vi "Do.vi"(8 "error in":errorcluster, 10 "Actor in":refnum<class "Actor.lvclass">, 11 "Update Device Config MSG":refnum<class "Update Device Config MSG.lvclass">) -> (0 "error out":errorcluster, 2 "Actor out":refnum<class "Actor.lvclass">)   [LabVIEW 2017, in "Controller.lvlib" / "Update Device Config MSG.lvclass"]
doc: "(<B>Filename</B>: Actor Framework.lvlib:Message.lvclass:Do.vi)\n\nDefines what a message does when it is received by an actor. Generally, a message instructs an actor to invoke one of its methods. By default, this method does nothing. A child class must override it to define behavior. Create a child class by using the Actor Framework Message Maker dialog box."
uses:
  Update Device Config MSG.lvclass
  C:/Program Files (x86)/National Instruments/LabVIEW 2017/vi.lib/MSR Consulting, LLC/Devices/DAQ Device/Messages/Device Configuration/Get Serialized Device Configuration MSG.lvclass
  <vilib>/ActorFramework/Actor/Actor.lvclass
  <vilib>/MSR Consulting, LLC/General Reuse/SuperActor/SuperActor.lvclass
  C:/Program Files (x86)/National Instruments/LabVIEW 2017/vi.lib/ActorFramework/Actor/Actor.lvclass
  <vilib>/MSR Consulting, LLC/Devices/DAQ Device/Messages/Device Configuration/Get Serialized Device Configuration MSG.lvclass/Get Serialized Device Configuration MSG.ctl
  <vilib>/MSR Consulting, LLC/General Reuse/SuperActor/SuperActor.lvclass/SuperActor.ctl
  <vilib>/MSR Consulting, LLC/Devices/DAQ Device/Messages/Device Configuration/Read cfg cluster.vi
  <vilib>/MSR Consulting, LLC/General Reuse/SuperActor/Read CVT Session.vi
  <vilib>/MSR Consulting, LLC/General Reuse/SuperActor/Read Log Session.vi
  <vilib>/MSR Consulting, LLC/General Reuse/Session APIs/_Session Fwk/Session - Root.lvclass
  <vilib>/MSR Consulting, LLC/General Reuse/Session APIs/CVT/CVT.lvclass
  <vilib>/MSR Consulting, LLC/General Reuse/Session APIs/Session Log/System Log.lvclass
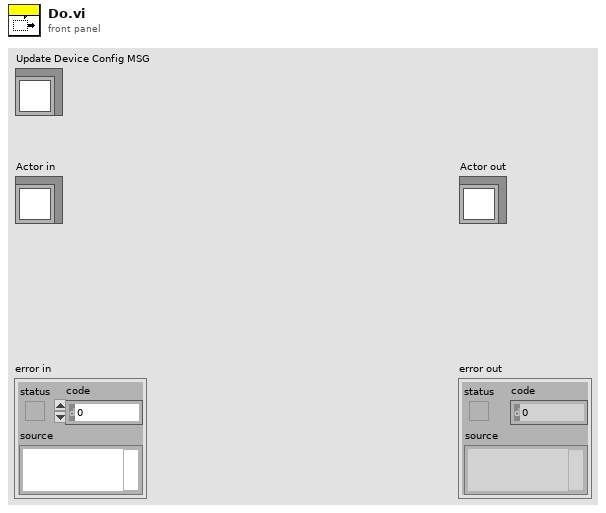
[diagram p1: front panel]
types:
  T1 = typedef "DAQ Device.lvlib/Cfg Msg.ctl" = cluster{"ID":string, "type":string, "label":string, "SN":string, "controller_":bool, "Addr":string, "Model":string, "Device Active":bool}
  T2 = typedef "Session - Root.lvclass/Session Handle.ctl" = refnum<data-value>
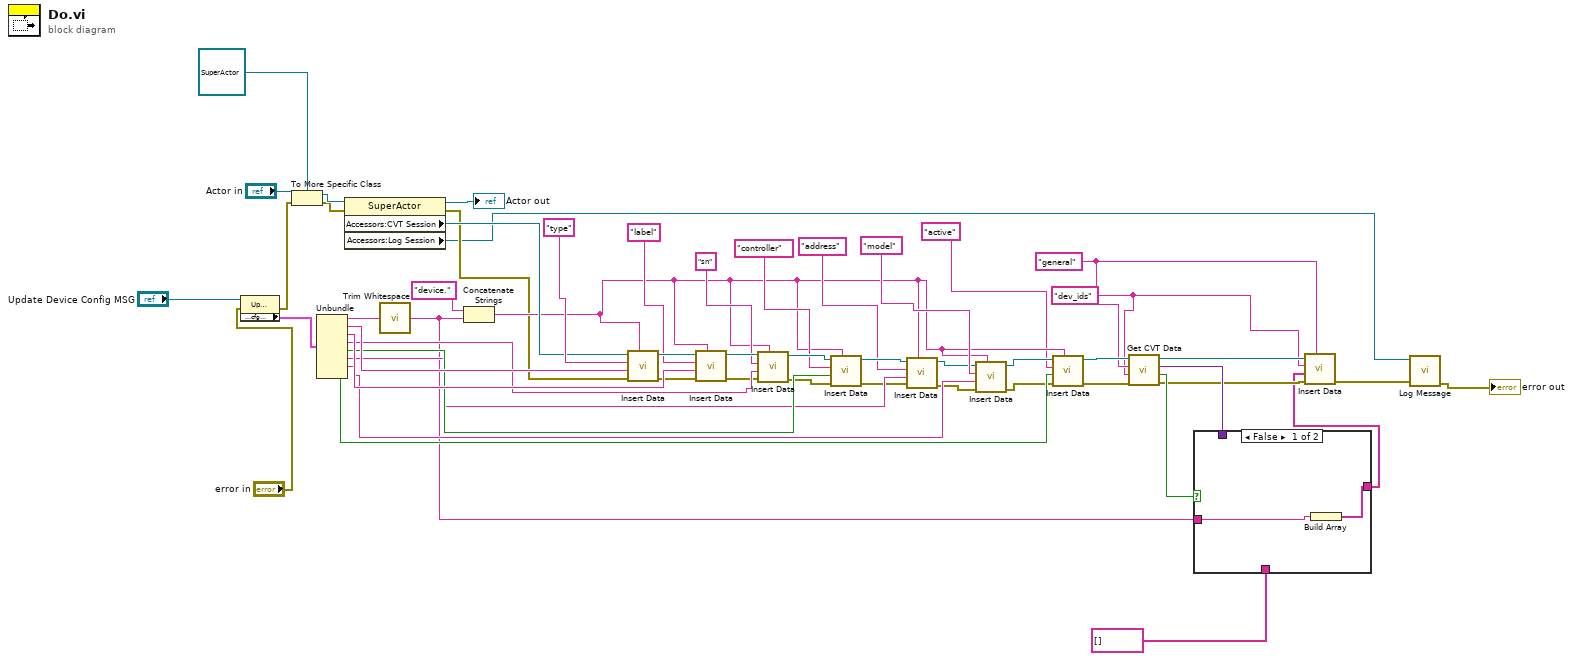
[diagram p0: block diagram]
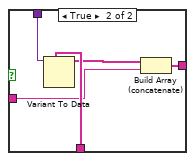
[diagram p2: hidden frame]
diagram:
  w2 = "general" ("Group")
  w1 = "dev_ids" ("Group")
  n1 = property class="Update Device Config MSG.lvclas"(reference="Update Device Config MSG", error in="error in") -> (error out=w23:errorcluster, "Accessors:cfg cluster"=w49:T1)  [unwired: 1 out]
  n2 = To More Specific Class(target class=refnum<class "SuperActor.lvclass"> refnum ("SuperActor.lvlib:SuperActor"), reference="Actor in", error in=w23) -> (specific class reference=w52:refnum<class "SuperActor.lvclass">, error out=w22:errorcluster)
  n3 = Unbundle(w49) -> ("ID"=w47:string, "type"=w44:string, "label"=w41:string, "SN"=w38:string, "controller_"=w35:bool, "Addr"=w32:string, "Model"=w29:string, "Device Active"=w25:bool)
  n4 = property class="SuperActor"(reference=w52, error in=w22) -> (reference out=→"Actor out":refnum<class "SuperActor.lvclass">, error out=w21:errorcluster, "Accessors:CVT Session"=w43:T2, "Accessors:Log Session"=w14:T2)
  n5 = call <vilib>:"Trim Whitespace.vi"("string"=w47) -> ("trimmed string"=w7:string)  [unwired: 1 in]
  n6 = Concatenate Strings("device." ("string"), w7) -> (w27:string)
  n7 = call <vilib>:"Insert Data.vi"("Group"=w27, "error in"=w21, "Data"=w44, "tag"="type", "CVT Session In"=w43) -> ("error out"=w20:errorcluster, "CVT Session Out"=w45:T2)  [unwired: 5 in]
  n8 = call <vilib>:"Insert Data.vi"("Group"=w27, "error in"=w20, "Data"=w41, "tag"="label", "CVT Session In"=w45) -> ("error out"=w19:errorcluster, "CVT Session Out"=w40:T2)  [unwired: 5 in]
  n9 = call <vilib>:"Insert Data.vi"("Group"=w27, "error in"=w19, "Data"=w38, "tag"="sn", "CVT Session In"=w40) -> ("error out"=w18:errorcluster, "CVT Session Out"=w37:T2)  [unwired: 5 in]
  n10 = call <vilib>:"Insert Data.vi"("Group"=w27, "error in"=w18, "Data"=w35, "tag"="controller", "CVT Session In"=w37) -> ("error out"=w17:errorcluster, "CVT Session Out"=w34:T2)  [unwired: 5 in]
  n11 = call <vilib>:"Insert Data.vi"("Group"=w27, "error in"=w17, "Data"=w32, "tag"="address", "CVT Session In"=w34) -> ("error out"=w16:errorcluster, "CVT Session Out"=w30:T2)  [unwired: 5 in]
  n12 = call <vilib>:"Insert Data.vi"("Group"=w27, "error in"=w16, "Data"=w29, "tag"="model", "CVT Session In"=w30) -> ("error out"=w15:errorcluster, "CVT Session Out"=w28:T2)  [unwired: 5 in]
  n13 = call <vilib>:"Insert Data.vi"("Group"=w27, "error in"=w15, "Data"=w25, "tag"="active", "CVT Session In"=w28) -> ("error out"=w11:errorcluster, "CVT Session Out"=w12:T2)  [unwired: 5 in]
  n14 = call <vilib>:"Get CVT Data.vi"("error in"=w11, "Variable"=w1, "Group"=w2, "CVT Session In"=w12) -> ("error out"=w5:errorcluster, "found"=w10:bool, "Data Out"=w9:variant, "CVT Session Out"=w6:T2)  [unwired: 4 in]
  n15 = case shown="False" w10 {
    tunnel: w9 -> [_ w61]
    tunnel: string[] [] -> [_ w60]
    tunnel: w7 -> [w56 w58]
    tunnel: [w55 w57] -> w4
    frame False {
      n16 = Build Array(w56) -> (w55:string[])
    }
    frame True {
      n17 = Variant To Data(type=w60, Variant=w61) -> (data=w59:string[])  [unwired: 1 in, 1 out]
      n18 = Build Array (concatenate)(w59, w58) -> (w57:string[])
    }
  }
  n19 = call <vilib>:"Insert Data.vi"("Group"=w2, "error in"=w5, "Data"=w4, "tag"=w1, "CVT Session In"=w6) -> ("error out"=w3:errorcluster)  [unwired: 5 in, 1 out]
  n20 = call <vilib>:"Log Message.vi"("error in"=w3, "session in"=w14) -> ("error out"=→"error out":errorcluster)  [unwired: 8 in, 1 out]
